vi "Read VIAnCfg XML.vi"(8 "error in (no error)":errorcluster, 11 "VIAnCfg XML Path":path) -> (0 "error out":errorcluster, 3 "VIA CFG Data":T1 {"Test Configuration"."Test Ranking" items=["Low", "Normal", "High"]})   [LabVIEW 2020]
uses:
  <vilib>/addons/analyzer/Typedefs/VIACFGExport.ctl
  <vilib>/addons/analyzer/_analyzerctrls.llb/VIAnCtl TestRanking.ctl
  <vilib>/addons/analyzer/_analyzerctrls.llb/VIAnCtl Config Control Value.ctl
  <vilib>/addons/analyzer/Typedefs/VIAn Error Description.ctl
  <vilib>/xml/Load XML File.vi
  <vilib>/xml/Close Reference(Node).vi
  <vilib>/xml/NI_XML.lvlib
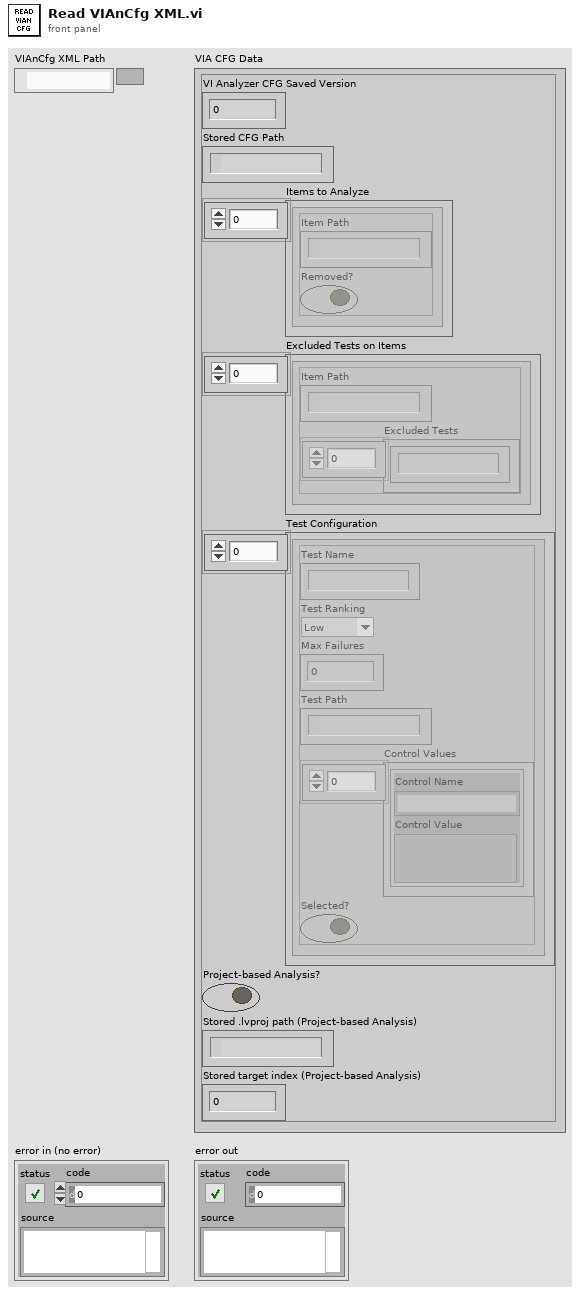
[diagram p1: front panel]
types:
  T1 = typedef "VIACFGExport.ctl" = cluster{"VI Analyzer CFG Saved Version":u16, "Stored CFG Path":path, "Items to Analyze":cluster{"Item Path":path, "Removed?":bool}[], "Excluded Tests on Items":cluster{"Item Path":path, "Excluded Tests":string[]}[], "Test Configuration":cluster{"Test Name":string, "Test Ranking":T2, "Max Failures":u32, "Test Path":path, "Control Values":T3[], "Selected?":bool}[], "Project-based Analysis?":bool, "Stored .lvproj path (Project-based Analysis)":path, "Stored target index (Project-based Analysis)":u16}
  T2 = typedef "VIAnCtl TestRanking.ctl" = u16
  T3 = typedef "VIAnCtl Config Control Value.ctl" = cluster{"Control Name":string, "Control Value":variant}
  T4 = typedef "VIAn Error Description.ctl" = enum16{"VIAnCfg Version Info", "VIAnalyzerConfiguration"}
  T5 = cluster{"VI Analyzer CFG Saved Version":u16, "StoredLvprojPath":string, "Project Based Analysis":bool}
  T6 = cluster{"Item Path":path, "Excluded Tests":string[]}[]
  T7 = cluster{"Test Name":string, "Test Ranking":T2, "Max Failures":u32, "Test Path":path, "Control Values":T3[], "Selected?":bool}[]
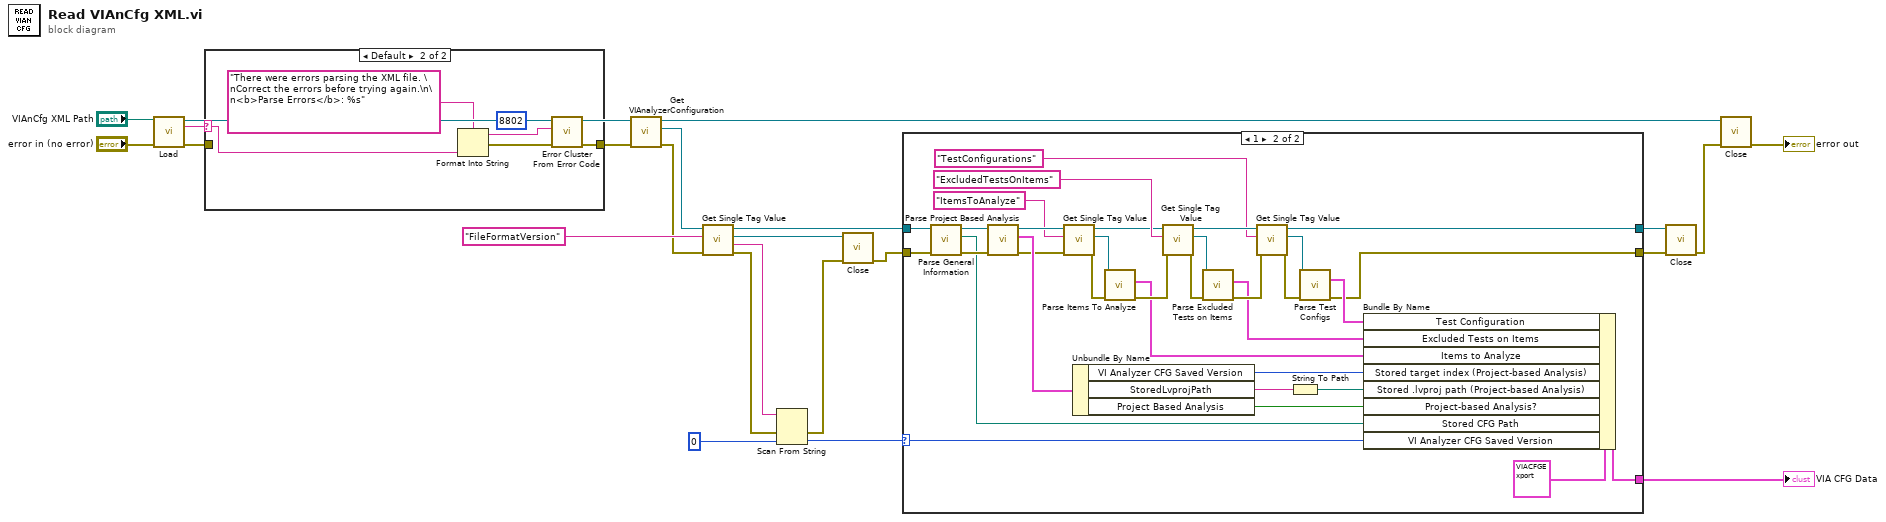
[diagram p0: block diagram]
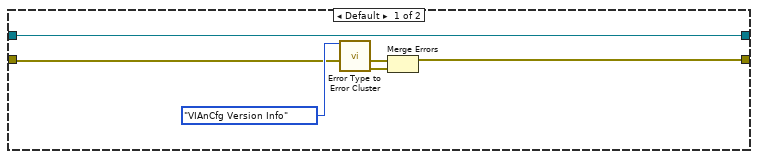
[diagram p3: hidden frame]
diagram:
  n1 = call-poly <vilib>:"Load.vi"("path to XML document"="VIAnCfg XML Path", "error in (no error)"="error in (no error)") -> ("DOM document out"=w17:refnum<k20>, "parse errors"=w21:string, "error out"=w22:errorcluster)  [unwired: 11 in]
  n2 = case shown="Default" w21 {
    selector: w21 -> [_ w27]
    tunnel: w22 -> [w24 _]
    tunnel: [w24 w25] -> w23
    frame "" {
    }
    frame Default {
      n3 = Format Into String(format string="There were errors parsing the XML file. \nCorrect the errors before trying again.\n\n<b>Parse Errors</b>: %s", w27) -> (resulting string=w28:string, error out=w26:errorcluster)  [unwired: 2 in]
      n4 = call <vilib>:"Error Cluster From Error Code.vi"("error in (no error)"=w26, "error message (\"\")"=w28, "error code (0)"=8802) -> ("error out"=w25:errorcluster)  [unwired: 6 in]
    }
  }
  n5 = call <vilib>:"Get VIAnalyzerConfiguration.vi"("error in"=w23, "DOM document in"=w17) -> ("error out"=w5:errorcluster, "Element"=w2:refnum<k20>, "DOM document out"=w12:refnum<k20>)  [unwired: 7 in]
  n6 = call <vilib>:"Get Single Tag Value.vi"("Error In"=w5, "Tag Name"="FileFormatVersion", "Element In"=w2) -> ("Error Out"=w9:errorcluster, "Tag Value"=w16:string, "Tag Reference"=w19:refnum<k20>, "Element Out"=w8:refnum<k20>)  [unwired: 5 in]
  n7 = Scan From String(input string=w16, error in=w9, default 1=u16 0 ("VI Analyzer CFG Saved Version")) -> (error out=w18:errorcluster, output 1=w7:u16)  [unwired: 2 in, 2 out]
  n8 = call-poly <vilib>:"Close.vi"("error in (no error)"=w18, "node"=w19) -> ("error out"=w20:errorcluster)  [unwired: 7 in]
  n9 = case shown="1" w7 {
    selector: w7 -> [_ w38]
    tunnel: w8 -> [w31 w68]
    tunnel: w20 -> [w33 w67]
    tunnel: [_ w64] -> w1
    tunnel: [w32 w62] -> w13
    tunnel: [w31 w51] -> w14
    frame Default {
      n10 = call <vilib>:"Error Type to Error Cluster.vi"("VIAn Error"=VIAn_Error_Description."VIAnCfg Version Info") -> ("error out"=w34:errorcluster)  [unwired: 14 in]
      n11 = Merge Errors(w33, w34) -> (w32:errorcluster)
    }
    frame 1 {
      n12 = call <vilib>:"Parse General Information.vi"("error in"=w67, "VIAnalyzerConfiguration in"=w68) -> ("error out"=w65:errorcluster, "StoredCFGPath"=w39:path, "VIAnalyzerConfiguration out"=w66:refnum<k20>)  [unwired: 7 in]
      n13 = call <vilib>:"Parse Project Based Analysis.vi"("error in (no error)"=w65, "Element in"=w66) -> ("error out"=w59:errorcluster, "Project Based Analysis"=w61:T5, "Element out"=w60:refnum<k20>)  [unwired: 7 in]
      n14 = call <vilib>:"Get Single Tag Value.vi"("Error In"=w59, "Tag Name"="ItemsToAnalyze", "Element In"=w60) -> ("Error Out"=w56:errorcluster, "Tag Reference"=w57:refnum<k20>, "Element Out"=w54:refnum<k20>)  [unwired: 5 in, 1 out]
      n15 = Unbundle By Name(w61) -> ("VI Analyzer CFG Saved Version"=w43:u16, "StoredLvprojPath"=w42:string, "Project Based Analysis"=w40:bool)
      n16 = call <vilib>:"Parse Items To Analyze.vi"("error in"=w56, "ItemsToAnalyze Element"=w57) -> ("error out"=w53:errorcluster, "Items To Analyze"=w44:cluster{"Item Path":path, "Removed?":bool}[])  [unwired: 8 in]
      n17 = call <vilib>:"Get Single Tag Value.vi"("Error In"=w53, "Tag Name"="ExcludedTestsOnItems", "Element In"=w54) -> ("Error Out"=w47:errorcluster, "Tag Reference"=w37:refnum<k20>, "Element Out"=w52:refnum<k20>)  [unwired: 5 in, 1 out]
      n18 = call <vilib>:"Parse Excluded Tests on Items.vi"("error in (no error)"=w47, "ExcludedTestsOnItems Element"=w37) -> ("error out"=w46:errorcluster, "Excluded Tests on Items"=w45:T6)  [unwired: 8 in]
      n19 = call <vilib>:"Get Single Tag Value.vi"("Error In"=w46, "Tag Name"="TestConfigurations", "Element In"=w52) -> ("Error Out"=w48:errorcluster, "Tag Reference"=w50:refnum<k20>, "Element Out"=w51:refnum<k20>)  [unwired: 5 in, 1 out]
      n20 = String To Path(string=w42) -> (path=w41:path)
      n21 = call <vilib>:"Parse Test Configs.vi"("TestConfigurations Element"=w50, "error in"=w48) -> ("Test Configurations"=w63:T7, "error out"=w62:errorcluster)  [unwired: 12 in]
      n22 = Bundle By Name(cluster=T1 {"VI Analyzer CFG Saved Version"=0, "Stored CFG Path"=path "", "Items to Analyze"=[], "Excluded Tests on Items"=[], "Test Configuration"=[], "Project-based Analysis?"=FALSE, "Stored .lvproj path (Project-based Analysis)"=path "", "Stored target index (Project-based Analysis)"=0} ("VIA CFG Data"), "Test Configuration"=w63, "Excluded Tests on Items"=w45, "Items to Analyze"=w44, "Stored target index (Project-based Analysis)"=w43, "Stored .lvproj path (Project-based Analysis)"=w41, "Project-based Analysis?"=w40, "Stored CFG Path"=w39, "VI Analyzer CFG Saved Version"=w38) -> (w64:T1)
    }
  }
  "VIA CFG Data" <- w1
  n23 = call-poly <vilib>:"Close.vi"("error in (no error)"=w13, "node"=w14) -> ("error out"=w15:errorcluster)  [unwired: 7 in]
  n24 = call-poly <vilib>:"Close.vi"("error in (no error)"=w15, "node"=w12) -> ("error out"=→"error out":errorcluster)  [unwired: 7 in]
